vi "lvEtherbone.socket_wait4Activity.vi"(0 "eb_socketID":i32, 3 "timeout [ms]":i32=10000, 5 "error in (no error)":errorcluster) -> (13 "eb_status_t":T2, 14 "eb_socketID out":i32, 15 "nRead":i32, 16 "nWrite":i32, 17 "timed out":bool, 18 "lastActivity":T1, 19 "error out":errorcluster)   [LabVIEW 2009, in "lvEtherbone.lvlib"]
doc: "//-----------------------------------------------------------------------------------\n// author : Dietrich Beck, GSI-Darmstadt\n// purpose : wait for activity on the Etherbone socket. This function MUST be called,\n// if a virtual device has been set up by using a handler\n// returns : lveb_status_t\n//-----------------------------------------------------------------------------------\nETHERBONE_API int lveb_socket_wait4Activity(int eb_socketID, //very important socket ID\n int timeout, //timeout [ms]\n int *lastActivity, //last activity on socket\n int *nRead, //nOf read cycles\n int *nWrite //nOf write cycles\n );"
uses:
  lvEtherbone.lvlib
  lvEtherbone.lveb_status_t.ctl
  lvEtherbone.lveb_activity_t.ctl
  bin/lvEtherbone.dll
panel:
  in  "myeb_activity_t":T1
  in  "myeb_status_t":T2
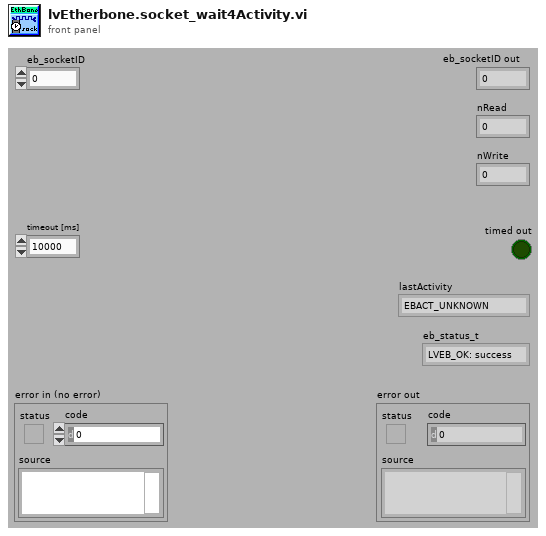
[diagram p1: front panel]
types:
  T1 = typedef "lvEtherbone.lvlib/lvEtherbone.lveb_activity_t.ctl" = enum32{"EBACT_UNKNOWN", "EBACT_TIMEDOUT", "EBACT_READ", "EBACT_WRITE", "EBACT_RW"}
  T2 = typedef "lvEtherbone.lvlib/lvEtherbone.lveb_status_t.ctl" = enum32{"LVEB_OK: success", "LVEB_UNKNOWN: unknown error", "LVEB_OS: operating system forbids access", "LVEB_PORT: port in use or unavailable", "LVEB_ID: ID invalid or out of resources", "LVEB_SOCKET: socket invalid or unavailable", "LVEB_EB: remote address is not Etherbone conformant", "LVEB_IP: bad format or network address", "LVEB_PORTWIDTH: port width error", "LVEB_DEVICEBUSY: Etherbone device still busy", "LVEB_DEVICEFAIL: operation on Wishbone device failed", "LVEB_DEVICEEXIST: Etherbone device already exists, overlaps, or does not exist", "LVEB_TIMEDOUT: a timeout occurred", "LVEB_OVERFLOW: payload of Etherbone exceeded", "LVEB_ADDRESS: bad address", "LVEB_ADDRESSWIDTH: address width error"}
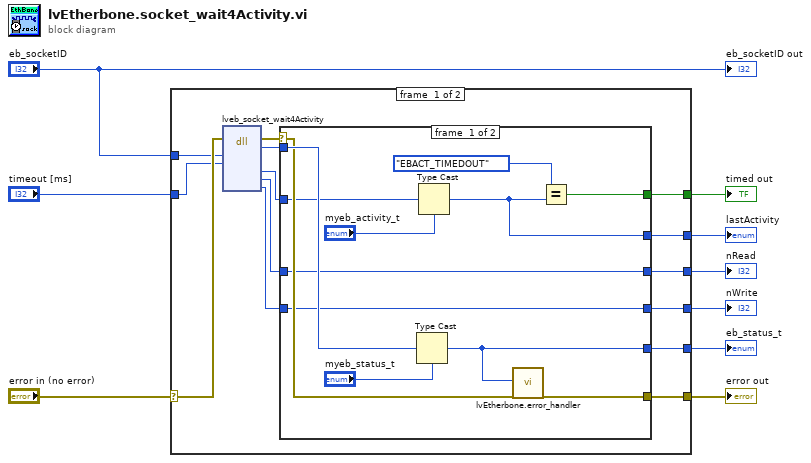
[diagram p0: block diagram]
diagram:
  n1 = case shown="No Error" "error in (no error)" {
    selector: "error in (no error)" -> [w23 w37]
    tunnel: [w19 w37] -> w8
    tunnel: "eb_socketID" -> [w22 _]
    tunnel: "timeout [ms]" -> [w21 _]
    tunnel: [w17 _] -> w5
    tunnel: [w16 _] -> w4
    tunnel: [w14 _] -> w3
    tunnel: [w12 _] -> w2
    tunnel: [w11 _] -> w1
    frame #0 {
      n2 = dll-call lib="F:/beck/Project/BEL/SCC/etherbone-core/api/lvEtherbone/bin/lvEtherbone.*" fn="lveb_socket_wait4Activity"(error in=w23, "eb_socketID"=w22, "timeout"=w21) -> (error out=w20:errorcluster, "myeb_status_t"=w18:i32, "lastActivity"=w15:i32, "nRead"=w13:i32, "nWrite"=w10:i32)  [unwired: 7 in, 1 out]
      n3 = case shown="No Error" w20 {
        selector: w20 -> [w31 w36]
        tunnel: w18 -> [w35 _]
        tunnel: [w33 _] -> w17
        tunnel: [w32 w36] -> w19
        tunnel: [w26 _] -> w16
        tunnel: w15 -> [w29 _]
        tunnel: [w28 _] -> w14
        tunnel: w13 -> [w25 _]
        tunnel: [w25 _] -> w12
        tunnel: [w24 _] -> w11
        tunnel: w10 -> [w24 _]
        frame #0 {
          n4 = Type Cast(type="myeb_status_t", x=w35) -> (*(type *) &x=w33:T2)
          n5 = Type Cast(type="myeb_activity_t", x=w29) -> (*(type *) &x=w28:T1)
          n6 = call "lvEtherbone.error_handler.vi"("eb_status"=w33, "error in"=w31) -> ("error out"=w32:errorcluster)  [unwired: 17 in]
          n7 = Equal?(x=lvEtherbone.lveb_activity_t."EBACT_TIMEDOUT", y=w28) -> (x = y?=w26:bool)
        }
        frame #1 {
        }
      }
    }
    frame #1 {
    }
  }
  "error out" <- w8
  "eb_status_t" <- w5
  "timed out" <- w4
  "lastActivity" <- w3
  "nRead" <- w2
  "nWrite" <- w1
  "eb_socketID out" <- "eb_socketID"
